vi "Globals.vi"() -> ()   [LabVIEW 2017, in "nifxpmath_Atan2.xnode"]
uses:
  <vilib>/rvi/FXPMathLib/FxpAtan2/XNode/nifxpmath_Atan2.xnode
panel:
  in  "Term Z Name w/o Unit":string="atan2(y,x)"
  out "Small Icon":picture
  in  "Term Z Name":string="atan2(y,x) (pi)"
  in  "Term Y Name":string="y"
  in  "Term X Name":string="x"
  in  "Term Z ID":string="TERM_XY"
  in  "Term Y ID":string="TERM_Y"
  in  "Term X ID":string="TERM_X"
  out "Normal Banner":picture
  out "Small Icon w/ 4Wire":picture
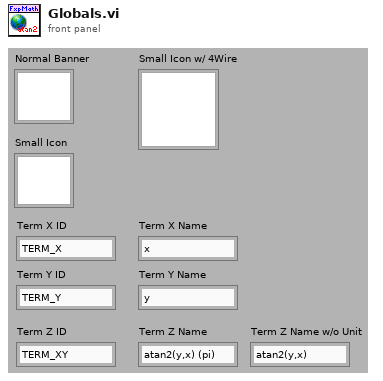
[diagram p1: front panel]
diagram:
